vi "Receive.vi"(8 "error in (no error)":errorcluster, 11 "Message Queue":refnum<queue>) -> (0 "error out":errorcluster, 1 "Result/Error":variant, 3 "Message":string, 4 "Exit":bool, 6 "Backlog":i32)   [LabVIEW 2020]
uses:
  Message Queue/Message Cluster.ctl
  Message Queue/Message Queue.lvlib
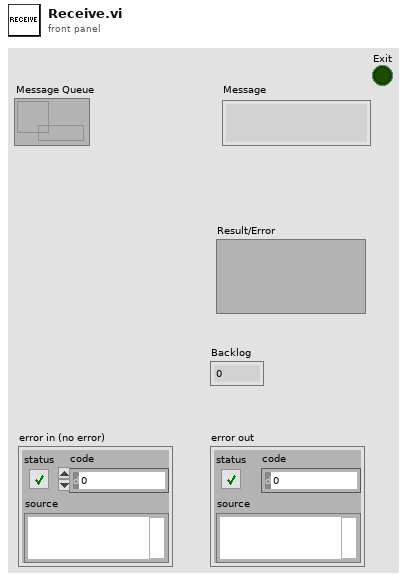
[diagram p1: front panel]
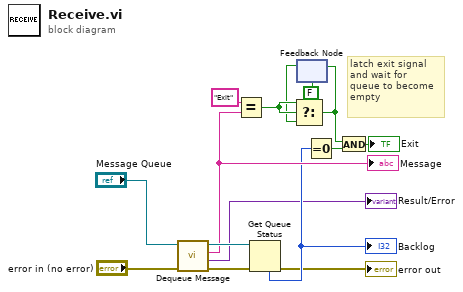
[diagram p0: block diagram]
diagram:
  # "latch exit signal\nand wait for\nqueue to become\nempty"
  n1 = call "Dequeue Message.vi"("error in (no error)"="error in (no error)", "Message Queue"="Message Queue") -> ("error out"=w12:errorcluster, "Message Data"=→"Result/Error":variant, "Message"=w11:string, "dup Message Queue"=w13:refnum<queue>)  [unwired: 6 in]
  "Message" <- w11
  n2 = Equal?(x="Exit", y=w11) -> (x = y?=w7:bool)
  n3 = Get Queue Status(queue=w13, error in (no error)=w12) -> (error out=→"error out":errorcluster, # elements in queue=w3:i32)  [unwired: 1 in, 6 out]
  "Backlog" <- w3
  n4 = feedback #1(FALSE) -> (w6:bool)
  n5 = Select(t=w7, s=w7, f=w6) -> (s? t:f=w4:bool)
  n6 = feedback-in #1(w4) -> ()
  n7 = Equal To 0?(x=w3) -> (x = 0?=w9:bool)
  n8 = And(x=w4, y=w9) -> (x .and. y?=→"Exit":bool)
